vi "Midi Note On.vi"(4 "Volume":i32, 5 "Note":i32, 6 "Channel":i32, 7 "MIDI handle":i32) -> (0 "Win32 error code":i32, 3 "Duplicate MIDI handle":i32)   [LabVIEW 2016]
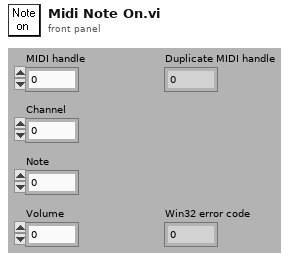
[diagram p1: front panel]
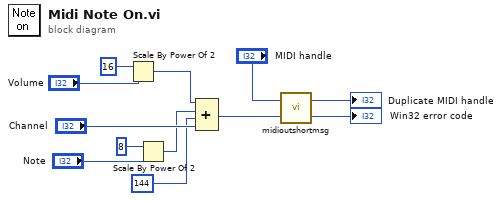
[diagram p0: block diagram]
diagram:
  n1 = Scale By Power Of 2(n=16, x="Volume") -> (x*2^n=w7:i32)
  n2 = Scale By Power Of 2(n=8, x="Note") -> (x*2^n=w9:i32)
  n3 = Compound Arithmetic op=ADD(w7, w9, 144 ("data"), "Channel") -> (w10:i32)
  n4 = call "midioutshortmsg.vi"("Data"=w10, "MIDI output handle"="MIDI handle") -> ("Win32 error code"=→"Win32 error code":i32, "Duplicate MIDI output handle"=→"Duplicate MIDI handle":i32)
